vi "GEA2 Read ERD Multiple Messages.vi"(0 "GEA2 Reference In":refnum<k24>, 1 "Retry Count":i32=5, 2 "Read Timeout (ms)":u32=500, 5 "GEA Inputs":T4 {"Destination" format="%.0x"; "Source" format="%.0x"}, 7 "Read ERD List":T2[](array[typedef]) {"ERD Number" format="%.0x"}, 9 "GEA2 Event Registration":refnum<event-registration>, 11 "Error In":errorcluster, 12 "#ERDs per message":i32=1 min=1 step=1, 13 "Verify ERD Response?":bool=TRUE) -> (4 "GEA2 Reference Out":refnum<k24>, 6 "Raw Data Out":string[](array[string]), 8 "ERD Data Out":T1[](array[typedef]) {"ERD Number" format="%.0x"}, 10 "Event Registration Refnum":refnum<event-registration>, 15 "Error Out":errorcluster)   [LabVIEW 2016, in "GEA2_Toolkit.lvlib"]
uses:
  library/GEA2_Toolkit.lvlib
  type defs/Source_Destination.ctl
  type defs/ERD Read Data In.ctl
  type defs/Data Type.ctl
  type defs/ERD Read Data Out.ctl
  C:/TechnologyLab/NI-2010/Trunk/Utility/LabVIEW GEA2 Toolkit v1.0.0.0/Appliance.NET/GeaCommunication.dll
  Appliance.NET/GeaCommunication.dll
  type defs/Data Out.ctl
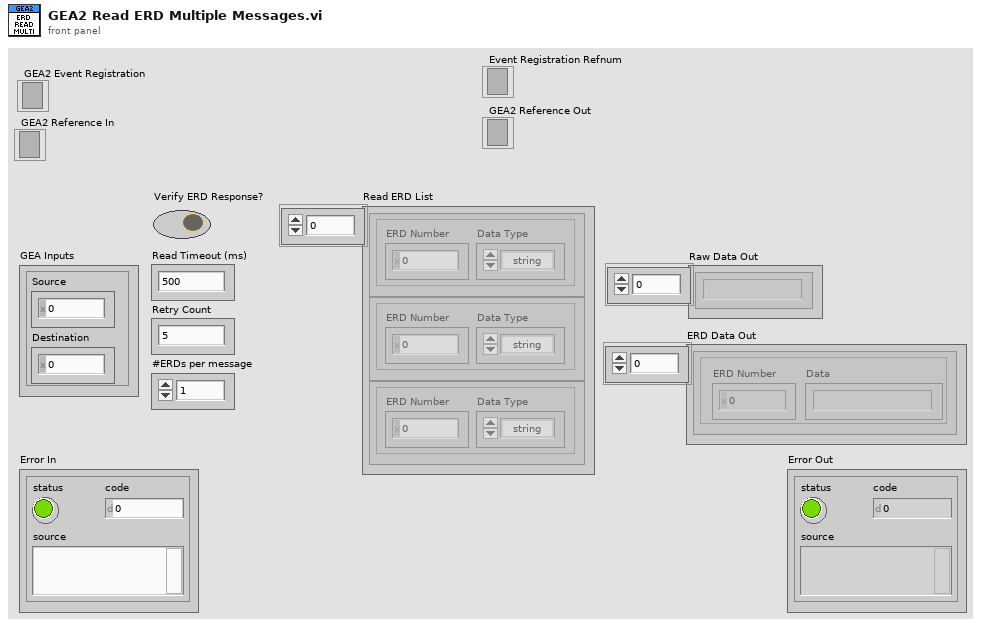
[diagram p1: front panel]
types:
  T1 = typedef "GEA2_Toolkit.lvlib/ERD Read Data Out.ctl" = cluster{"ERD Number":u16, "Data":string}
  T2 = typedef "GEA2_Toolkit.lvlib/ERD Read Data In.ctl" = cluster{"ERD Number":u16, "Data Type":T3}
  T3 = typedef "GEA2_Toolkit.lvlib/Data Type.ctl" = enum16{"string", "boolean", "uint8_t", "uint16_t", "uint32_t", "uint64_t"}
  T4 = typedef "GEA2_Toolkit.lvlib/Source_Destination.ctl" = cluster{"Source":u8, "Destination":u8}
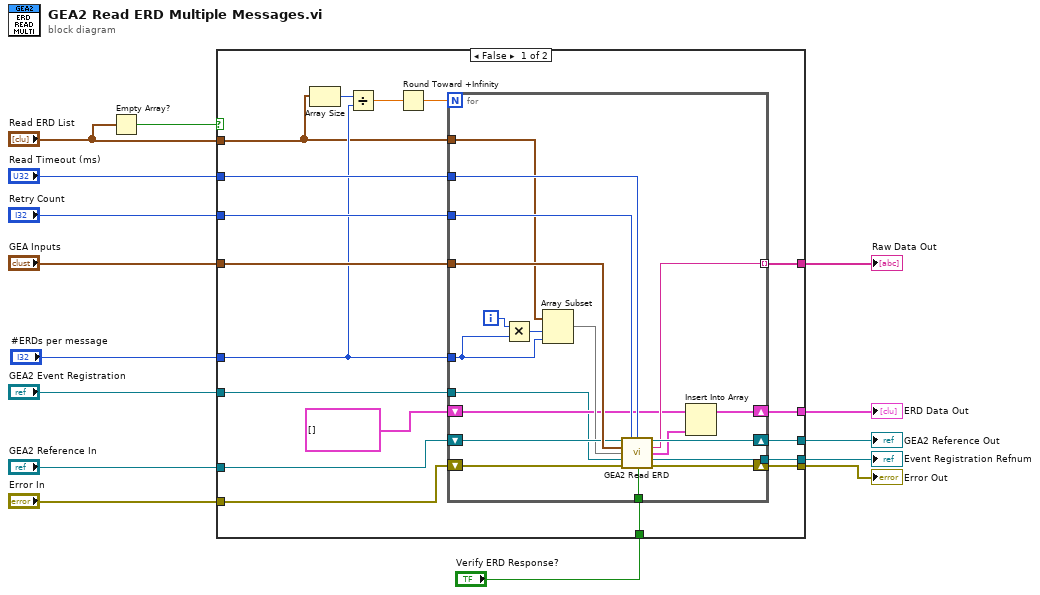
[diagram p0: block diagram]
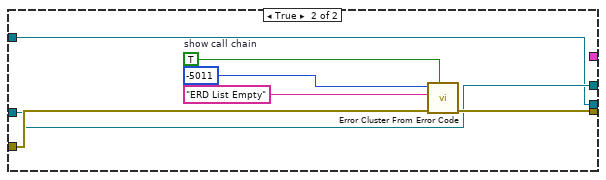
[diagram p2: hidden frame]
diagram:
  n1 = Empty Array?(array="Read ERD List") -> (empty?=w5:bool)
  n2 = case shown="False" w5 {
    tunnel: [w33 w54] -> w3
    tunnel: "Error In" -> [w32 w56]
    tunnel: [w31 w55] -> w14
    tunnel: "Verify ERD Response?" -> [w30 _]
    tunnel: "GEA Inputs" -> [w29 _]
    tunnel: "Read Timeout (ms)" -> [w28 _]
    tunnel: "Retry Count" -> [w27 _]
    tunnel: "GEA2 Reference In" -> [w26 w54]
    tunnel: "#ERDs per message" -> [w22 _]
    tunnel: [w21 _] -> w8
    tunnel: [w19 _] -> w7
    tunnel: "Read ERD List" -> [w18 _]
    tunnel: "GEA2 Event Registration" -> [w17 w53]
    tunnel: [w16 w53] -> w1
    frame False {
      n3 = Array Size(array=w18) -> (size(s)=w25:i32)
      n4 = Divide(x=w25, y=w22) -> (x/y=w24:dbl)
      n5 = Round Toward +Infinity(x=w24) -> (ceil(x): smallest int >= x=w23:dbl)
      n6 = for {
        N: w23 -> [_]
        tunnel: w30 -> [w49]
        tunnel: w29 -> [w48]
        tunnel: [w47] -> w21 mode=indexing
        tunnel: w28 -> [w46]
        tunnel: w27 -> [w45]
        shift-right: [w52] -> w33
        shift-left: w26 -> [w40]
        shift-right: [w50] -> w31
        shift-left: w32 -> [w51]
        tunnel: w18 -> [w44]
        tunnel: w22 -> [w43]
        shift-right: [w36] -> w19
        shift-left: T1[] [] -> [w38]
        tunnel: w17 -> [w35]
        tunnel: [w34] -> w16
        i -> [w42]
        n7 = Multiply(x=w42, y=w43) -> (x*y=w41:i32)
        n8 = Array Subset(array=w44, index=w41, length=w43) -> (w39:T2[])
        n9 = call "GEA2 Read ERD.vi"("GEA2 Reference In"=w40, "Retry Count"=w45, "Read Timeout (ms)"=w46, "GEA Inputs"=w48, "Read ERD List"=w39, "GEA2 Event Registration"=w35, "Error In"=w51, "Verify ERD Response?"=w49) -> ("GEA2 Reference Out"=w52:refnum<k24>, "Raw Data Out"=w47:string, "ERD Data Out"=w37:T1[], "Event Registration Refnum"=w34:refnum<event-registration>, "Error Out"=w50:errorcluster)  [unwired: 3 in]
        n10 = Insert Into Array(array=w38, new element=w37) -> (w36:T1[])  [unwired: 1 in]
      }
    }
    frame True {
      w57 = TRUE  # show call chain
      n11 = call <vilib>:"Error Cluster From Error Code.vi"("show call chain? (False)"=w57, "error in (no error)"=w56, "error message (\"\")"="ERD List Empty" ("error message (\"\")"), "error code (0)"=-5011) -> ("error out"=w55:errorcluster)  [unwired: 5 in]
    }
  }
  "Error Out" <- w14
  "Raw Data Out" <- w8
  "ERD Data Out" <- w7
  "GEA2 Reference Out" <- w3
  "Event Registration Refnum" <- w1
